vi "Network adapter fetcher.vi"(7 "Match Exactly?":bool, 8 "error in (no error)":errorcluster, 9 "Filter Disconnected":bool, 10 "Filter dashes?":bool, 11 "Specific Connection":string="Ethernet") -> (0 "error out":errorcluster, 3 "Array":T1[](array[typedef]))   [LabVIEW 2020]
doc: "This VI calls a Windows shell command that fetches details of the installed Network Interface Cards. It then searches for valid Physical (MAC) Addresses and populates an array. If \"All adapters\" is set to True, then the whole array will be output. otherwise, only the first element will be output, which should correspond to the primary ethernet adapter."
uses:
  <vilib>/regexp/Match Regular Expression.xnode
  TypeDef/Network adaptor details.ctl
panel:
  out "Full Array":string[][](array[string])
  out "First Matched MAC":string
  out "Specific Connection":string[][](array[string])
  out "Connected Array":string[][](array[string])
  out "Shell Output":string
  # "Network card MAC Address Fetcher"
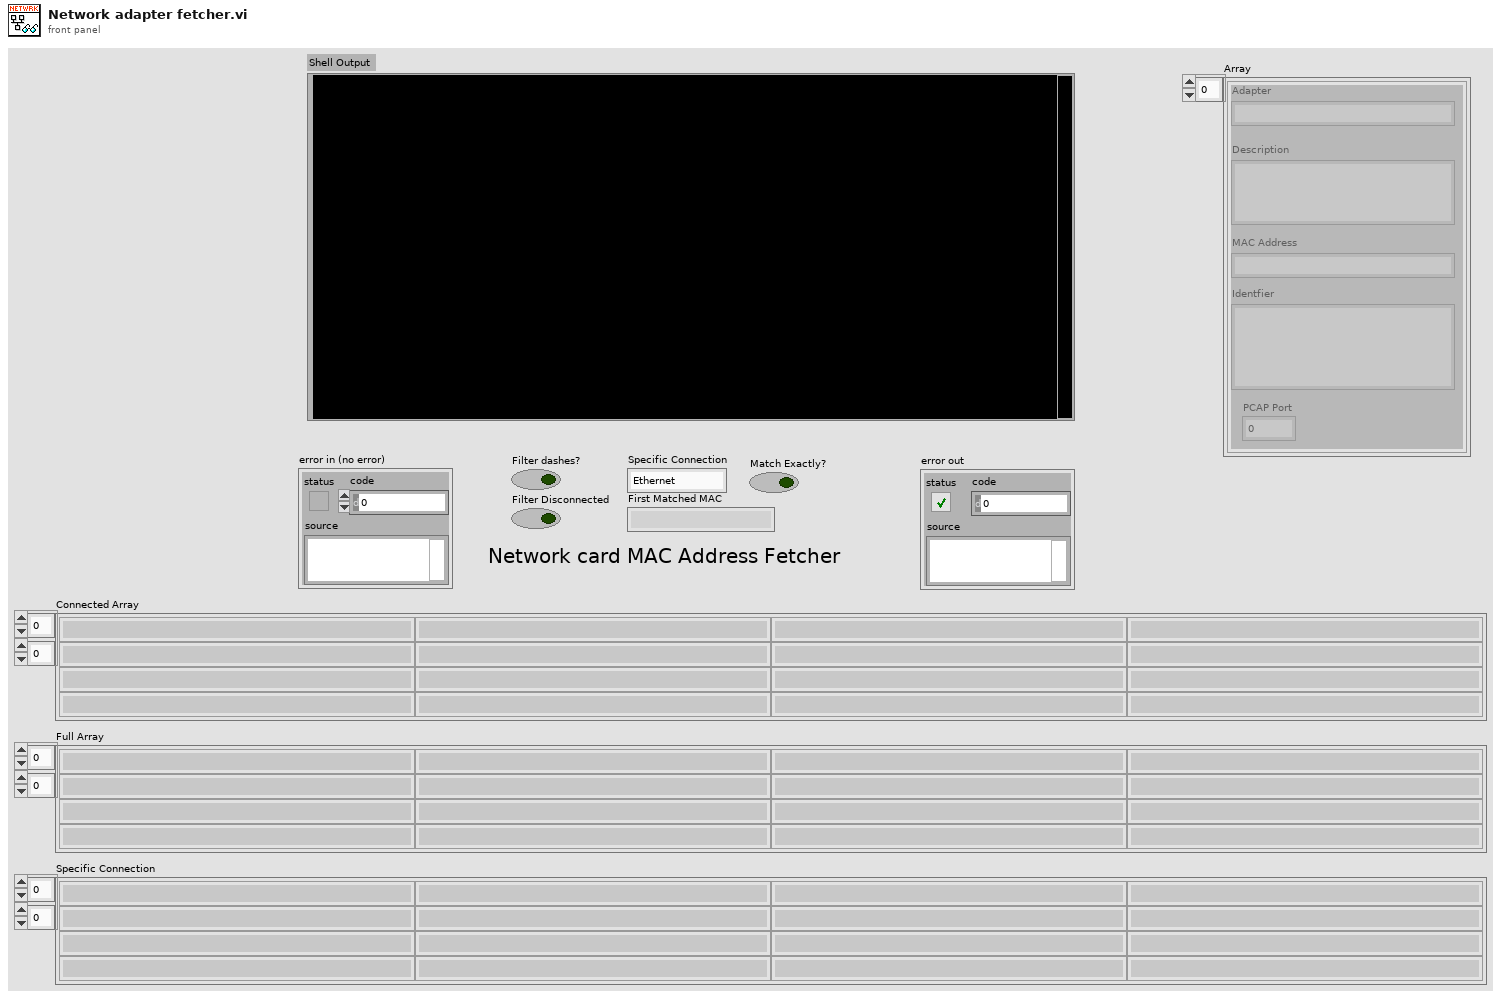
[diagram p1: front panel]
types:
  T1 = typedef "Network adaptor details.ctl" = cluster{"Adapter":string, "Description":string, "MAC Address":string, "Identfier":string, "PCAP Port":u32}
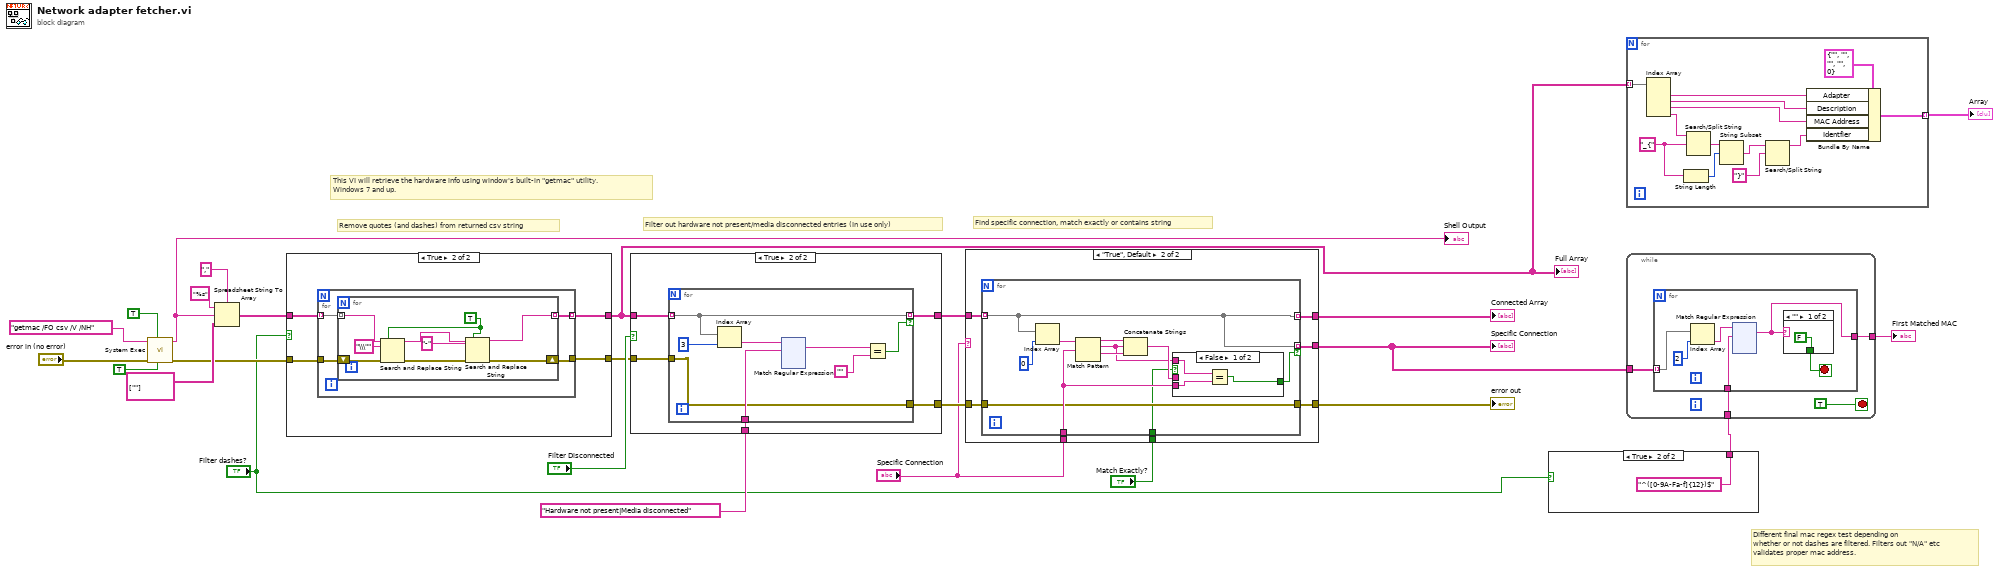
[diagram p0: block diagram]
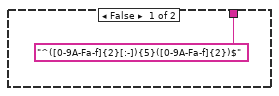
[diagram p2: hidden frame]
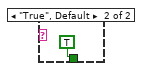
[diagram p3: hidden frame]
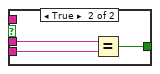
[diagram p5: hidden frame]
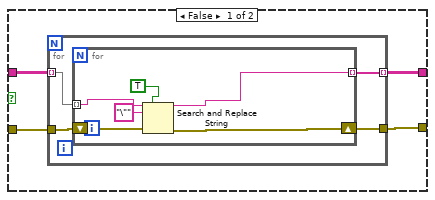
[diagram p7: hidden frame]
diagram:
  # "Different final mac regex test depending on\nwhether or not dashes are filtered. Filters out \"N/A\" etc\nvalidates proper mac address."
  # "Find specific connection, match exactly or contains string"
  # "Filter out hardware not present/media disconnected entries (In use only)"
  # "Remove quotes (and dashes) from returned csv string"
  # "This VI will retrieve the hardware info using window's built-in \"getmac\" utility.\nWindows 7 and up."
  n1 = call <vilib>:"System Exec.vi"("run minimized? (F)"=TRUE, "wait until completion? (T)"=TRUE ("run minimized? (F)"), "error in (no error)"="error in (no error)", "command line"="getmac /FO csv /V /NH") -> ("error out"=w13:errorcluster, "standard output"=w18:string)  [unwired: 4 in, 2 out]
  "Shell Output" <- w18
  n2 = Spreadsheet String To Array(delimiter (Tab)=",", format string="%s", spreadsheet string=w18, array type (2D Dbl)=string[][] [[""]]) -> (array=w14:string[][])
  n3 = case shown="True" "Filter dashes?" {
    tunnel: w13 -> [w29 w41]
    tunnel: [w28 w40] -> w12
    tunnel: w14 -> [w26 w43]
    tunnel: [w27 w42] -> w3
    frame False {
      n4 = for {
        tunnel: w29 -> [w33]
        tunnel: [w32] -> w28
        tunnel: [w30] -> w27 mode=indexing
        tunnel: w26 -> [w31] mode=indexing
        n5 = for {
          tunnel: w31 -> [w37] mode=indexing
          tunnel: [w34] -> w30 mode=indexing
          shift-right: [w35] -> w32
          shift-left: w33 -> [w38]
          n6 = Search and Replace String(replace all?=TRUE, input string=w37, search string="\"", error in=w38) -> (result string=w34:string, error out=w35:errorcluster)  [unwired: 4 in, 2 out]
        }
      }
    }
    frame True {
      n7 = for {
        tunnel: w43 -> [w46] mode=indexing
        tunnel: [w44] -> w42 mode=indexing
        tunnel: w41 -> [w47]
        tunnel: [w45] -> w40
        n8 = for {
          tunnel: w46 -> [w53] mode=indexing
          tunnel: [w49] -> w44 mode=indexing
          shift-right: [w48] -> w45
          shift-left: w47 -> [w55]
          w50 = TRUE ("replace all? (F)")
          n9 = Search and Replace String(replace all?=w50, input string=w53, search string="\\\"", error in=w55) -> (result string=w52:string, error out=w54:errorcluster)  [unwired: 4 in, 2 out]
          n10 = Search and Replace String(replace all?=w50, input string=w52, search string="-", error in=w54) -> (result string=w49:string, error out=w48:errorcluster)  [unwired: 4 in, 2 out]
        }
      }
    }
  }
  "Full Array" <- w3
  n11 = case shown="True" "Filter Disconnected" {
    tunnel: [w58 w62] -> w11
    tunnel: [w57 w59] -> w10
    tunnel: w3 -> [w57 w61]
    tunnel: w12 -> [w58 w63]
    tunnel: "Hardware not present|Media disconnected" -> [_ w60]
    frame False {
    }
    frame True {
      n12 = for {
        tunnel: w63 -> [w64]
        tunnel: w61 -> [w68] mode=indexing
        tunnel: w60 -> [w70]
        tunnel: [w68] -> w59 mode=indexing if=w69
        tunnel: [w64] -> w62
        n13 = Index Array(array=w68, index=3) -> (element=w67:string)
        n14 = xnode "Match Regular Expression"("input string"=w67, "regular expression"=w70) -> ("whole match"=w66:string)  [unwired: 4 in, 4 out]
        n15 = Equal?(x=w66, y="") -> (x = y?=w69:bool)
      }
    }
  }
  n16 = case shown="\"True\", Default" "Specific Connection" {
    tunnel: "Specific Connection" -> [_ w194]
    tunnel: [w187 w193] -> w20
    tunnel: [w187 w192] -> w7
    tunnel: [w186 w191] -> w19
    tunnel: w11 -> [w186 w190]
    tunnel: w10 -> [w187 w189]
    tunnel: "Match Exactly?" -> [_ w188]
    frame "" {
    }
    frame "True", Default {
      n17 = for {
        tunnel: w190 -> [w197]
        tunnel: w189 -> [w201] mode=indexing
        tunnel: w194 -> [w203]
        tunnel: [w201] -> w193 mode=indexing
        tunnel: [w201] -> w192 mode=indexing if=w202
        tunnel: [w197] -> w191
        tunnel: w188 -> [w196]
        n18 = Index Array(array=w201, index=0) -> (element=w204:string)
        n19 = Match Pattern(string=w204, regular expression=w203) -> (before substring=w200:string, match substring=w195:string, after substring=w199:string)  [unwired: 1 in, 1 out]
        n20 = Concatenate Strings(w200, w195, w199) -> (w198:string)
        n21 = case shown="False" w196 {
          tunnel: w203 -> [w207 w211]
          tunnel: [w206 w210] -> w202
          tunnel: w198 -> [_ w209]
          tunnel: w195 -> [w208 _]
          frame False {
            n22 = Equal?(x=w208, y=w207) -> (x = y?=w206:bool)
          }
          frame True {
            n23 = Equal?(x=w209, y=w211) -> (x = y?=w210:bool)
          }
        }
      }
    }
  }
  "Connected Array" <- w20
  "Specific Connection" <- w7
  "error out" <- w19
  n24 = case shown="True" "Filter dashes?" {
    tunnel: ["^([0-9A-Fa-f]{2}[:-]){5}([0-9A-Fa-f]{2})$" ("regular expression") "^([0-9A-Fa-f]{12})$" ("regular expression")] -> w4
    frame False {
    }
    frame True {
    }
  }
  n25 = for {
    tunnel: w3 -> [w225] mode=indexing
    tunnel: [w221] -> w2 mode=indexing
    w219 = "_{" ("search string/char (-)")
    n26 = Index Array(array=w225) -> (element #1=w224:string, element #2=w223:string, element #3=w222:string, element #4=w220:string)  [unwired: 4 in]
    n27 = String Length(string=w219) -> (length=w216:i32)
    n28 = Search/Split String(string=w220, search string/char (-)=w219) -> (match + rest of string=w217:string)  [unwired: 1 in, 2 out]
    n29 = String Subset(string=w217, offset (0)=w216) -> (substring=w215:string)  [unwired: 1 in]
    n30 = Search/Split String(string=w215, search string/char (-)="}") -> (substring before match=w218:string)  [unwired: 1 in, 2 out]
    n31 = Bundle By Name(cluster=T1 {"Adapter"="", "Description"="", "MAC Address"="", "Identfier"="", "PCAP Port"=0} ("Network Adapter details"), "Adapter"=w224, "Description"=w223, "MAC Address"=w222, "Identfier"=w218) -> (w221:T1)
  }
  "Array" <- w2
  n32 = while {
    tunnel: w7 -> [w230]
    tunnel: [w229] -> w6
    tunnel: w4 -> [w227]
    stop <- TRUE stop-if-true
    n33 = for {
      tunnel: w230 -> [w236] mode=indexing
      tunnel: [w232] -> w229
      tunnel: w227 -> [w231]
      stop <- w233 stop-if-true
      n34 = Index Array(array=w236, index=2 ("disabled index (col)")) -> (element=w234:string)
      n35 = xnode "Match Regular Expression"("input string"=w234, "regular expression"=w231) -> ("whole match"=w232:string)  [unwired: 4 in, 4 out]
      n36 = case shown="\"\"" w232 {
        tunnel: [FALSE TRUE] -> w233
        frame "" {
        }
        frame "True", Default {
        }
      }
    }
  }
  "First Matched MAC" <- w6
